vi "Test Decimator with State.vi"() -> ()   [LabVIEW 2019, in "DSP.lvclass"]
uses:
  DSP.lvclass
  Decimate DFD (Array).vi/949379ad-8373-41eb-be01-93a6c1c1afb3.vi
  Decimate DFD (Array).vi/efb08f77-0c38-4651-8a9c-351b9595fc15.vi
  <vilib>/addons/_JKI Toolkits/Caraya/classes/Assert/Assert Equal Value_Variant.vi
  <vilib>/addons/_JKI Toolkits/Caraya/classes/Assert/Assert.lvclass
  <vilib>/addons/_JKI Toolkits/Caraya/classes/Test/Test.lvclass
panel:
  out "Y":dbl[](array[numeric])
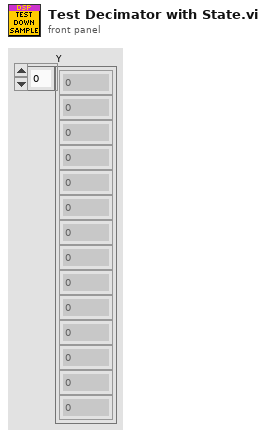
[diagram p1: front panel]
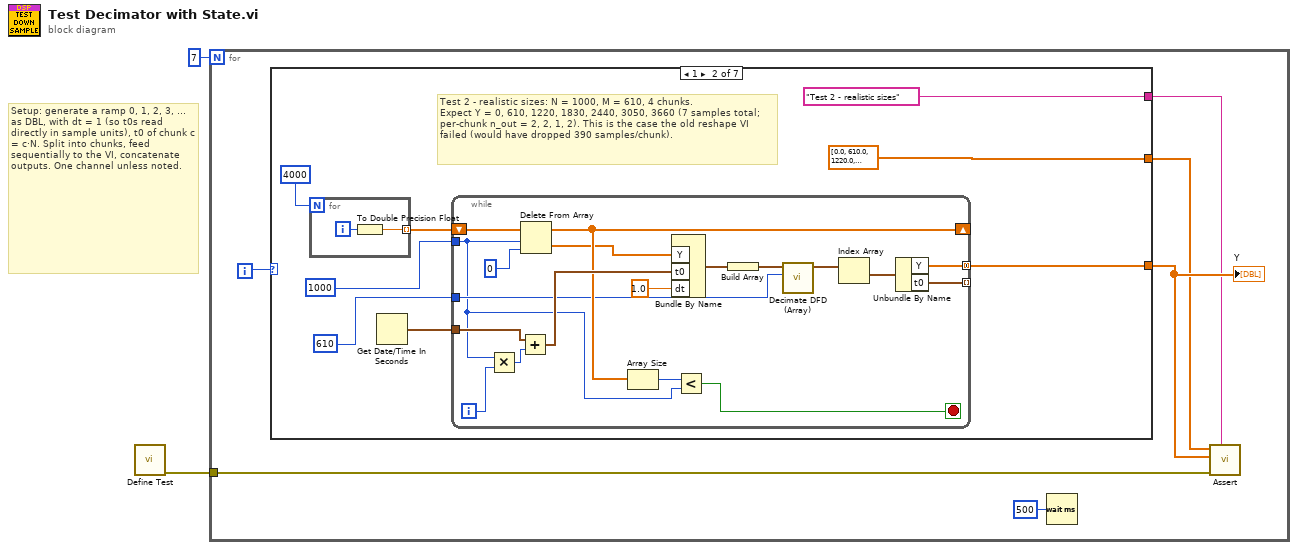
[diagram p0: block diagram]
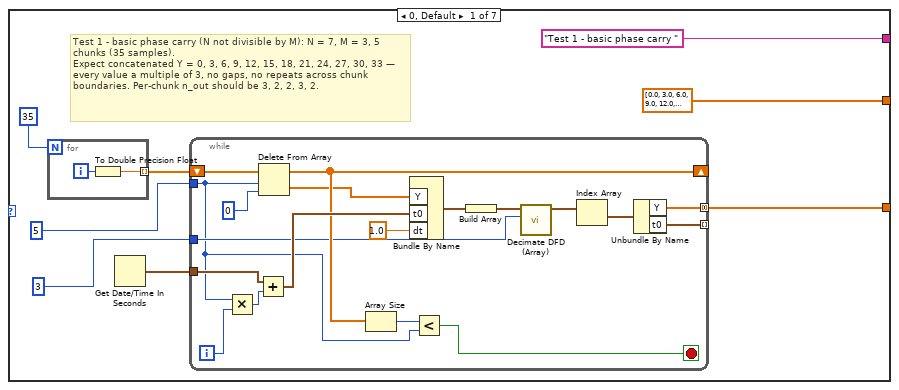
[diagram p2: hidden frame]
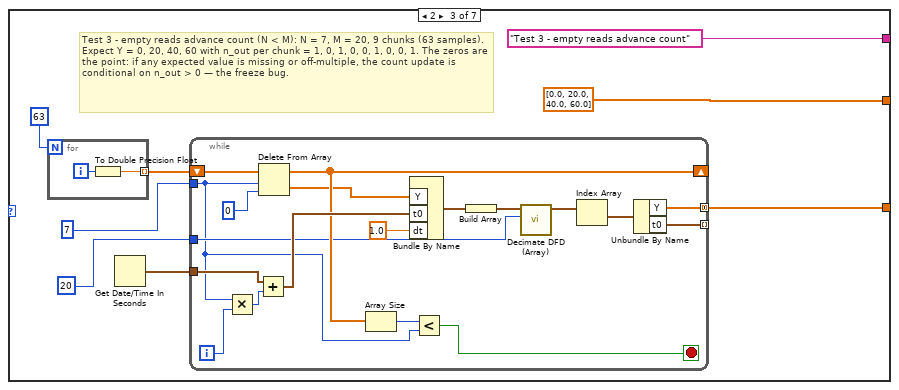
[diagram p3: hidden frame]
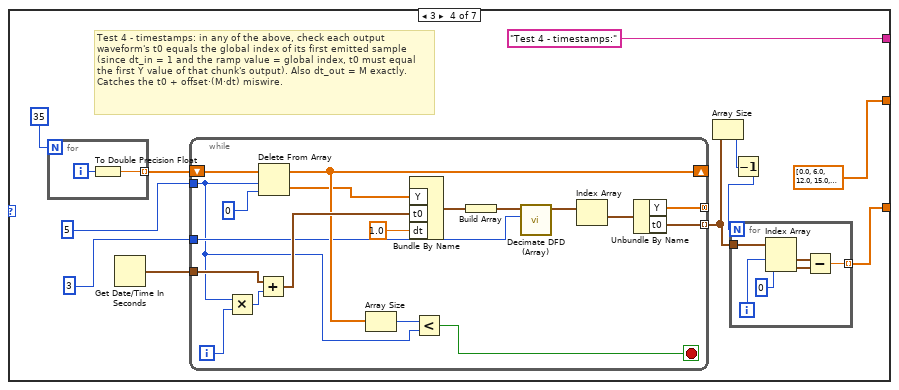
[diagram p4: hidden frame]
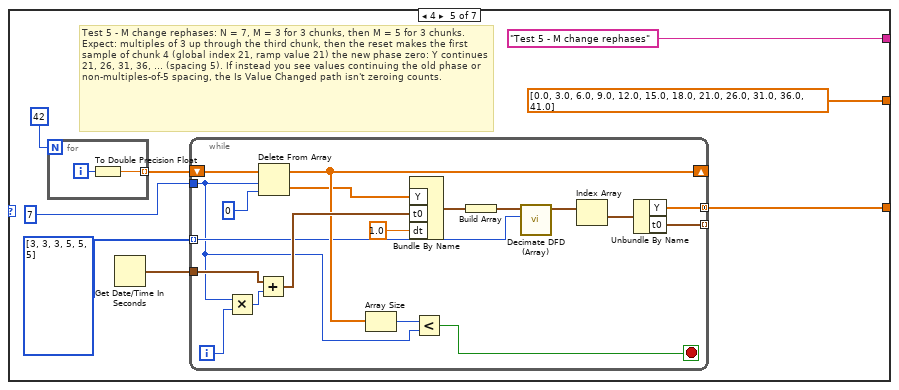
[diagram p5: hidden frame]
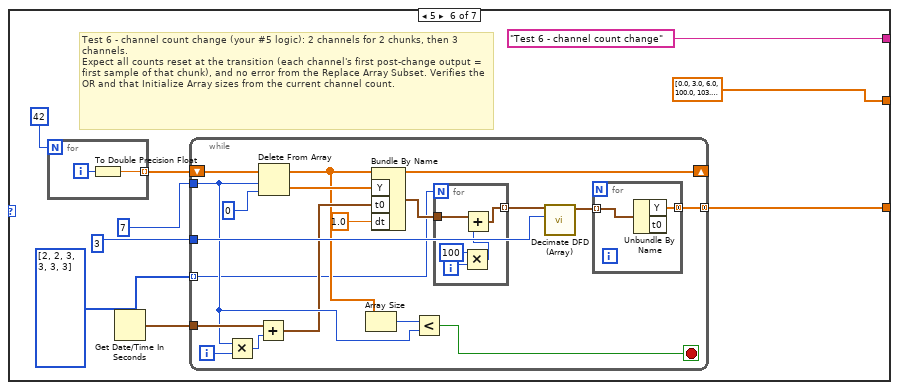
[diagram p6: hidden frame]
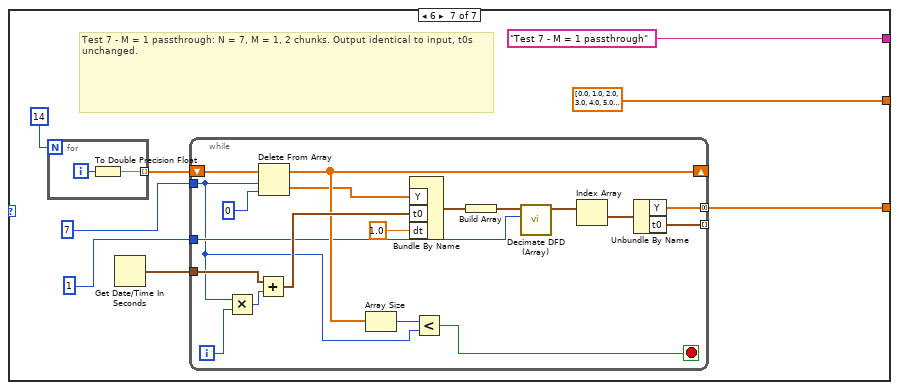
[diagram p7: hidden frame]
diagram:
  # "Setup: generate a ramp 0, 1, 2, 3, … as DBL, with dt = 1 (so t0s read directly in sample units), t0 of chunk c = c·N. Split into chunks, feed sequentially to the VI, concatenate outputs. One channel unless noted."
  n1 = call <vilib>:"Define Test.vi"() -> ("error out"=w1:errorcluster)  [unwired: 10 in, 1 out]
  n2 = for {
    N: 7 -> [_]
    tunnel: w1 -> [w4]
    i -> [w8]
    n3 = case shown="1" w8 {
      tunnel: [w16 w45 w74 w96 w141 w163 w206] -> w7
      tunnel: [dbl[] [0.0, 3.0, 6.0, 9.0, 12.0, 15.0, 18.0, 21.0, 24.0, 27.0, 30.0, 33.0] ("Y 2") dbl[] [0.0, 610.0, 1220.0, 1830.0, 2440.0, 3050.0, 3660.0] ("Y 2") dbl[] [0.0, 20.0, 40.0, 60.0] ("Y 2") dbl[] [0.0, 6.0, 12.0, 15.0, 21.0, 27.0] ("Array 2") dbl[] [0.0, 3.0, 6.0, 9.0, 12.0, 15.0, 18.0, 21.0, 26.0, 31.0, 36.0, 41.0] ("Y 2") dbl[] [0.0, 3.0, 6.0, 100.0, 103.0, 106.0, 9.0, 12.0, 109.0, 112.0, 14.0, 17.0, 20.0, 114.0, 117.0, 120.0, 214.0, 217.0, 220.0, 23.0, 26.0, 123.0, 126.0, 223.0, 226.0, 29.0, 32.0, 129.0, 132.0, 229.0, 232.0, 35.0, 38.0, 41.0, 135.0, 138.0, 141.0, 235.0, 238.0, 241.0] ("Y 3") dbl[] [0.0, 1.0, 2.0, 3.0, 4.0, 5.0, 6.0, 7.0, 8.0, 9.0, 10.0, 11.0, 12.0, 13.0] ("Y 2")] -> w6
      tunnel: ["Test 1 - basic phase carry " "Test 2 - realistic sizes" "Test 3 - empty reads advance count" "Test 4 - timestamps:" "Test 5 - M change rephases" "Test 6 - channel count change" "Test 7 - M = 1 passthrough"] -> w5
      frame 0, Default {
        # "Test 1 - basic phase carry (N not divisible by M): N = 7, M = 3, 5 chunks (35 samples).\nExpect concatenated Y = 0, 3, 6, 9, 12, 15, 18, 21, 24, 27, 30, 33 — every value a multiple of 3, no gaps, no repeats across chunk boundaries. Per-chunk n_out should be 3, 2, 2, 3, 2."
        n4 = for {
          N: 35 ("samples") -> [_]
          tunnel: [w36] -> w15 mode=indexing
          i -> [w37]
          n5 = To Double Precision Float(number=w37) -> (double precision float=w36:dbl)
        }
        n6 = Get Date/Time In Seconds() -> (seconds since 1Jan1904=w14:timestamp)
        n7 = while {
          tunnel: [w32] -> w16 mode=concatenating
          shift-right: [w21] -> _
          shift-left: w15 -> [w30]
          tunnel: 5 ("N") -> [w17]
          tunnel: w14 -> [w23]
          tunnel: 3 ("M") -> [w19]
          tunnel: [w18] -> _ mode=indexing
          i -> [w25]
          stop <- w27 stop-if-true
          n8 = Multiply(x=w17, y=w25) -> (x*y=w24:i32)
          n9 = Add(x=w23, y=w24) -> (x+y=w22:timestamp)
          n10 = Delete From Array(array=w30, length=w17, index=0) -> (deleted portion=w20:dbl[], array with subset deleted=w21:dbl[])
          n11 = Array Size(array=w21) -> (size(s)=w28:i32)
          n12 = Bundle By Name("Y"=w20, "t0"=w22, "dt"=1.0) -> (w26:waveform(dbl))  [unwired: 1 in]
          n13 = Less?(x=w28, y=w17) -> (x < y?=w27:bool)
          n14 = Build Array(w26) -> (w35:waveform(dbl)[])
          n15 = call "Decimate DFD (Array).vi"("Decimation Factor"=w19, "Waveforms in"=w35) -> ("waveforms out"=w34:waveform(dbl)[])  [unwired: 8 in, 1 out]
          n16 = Index Array(array=w34) -> (element=w33:waveform(dbl))  [unwired: 1 in]
          n17 = Unbundle By Name(w33) -> ("Y"=w32:dbl[], "t0"=w18:timestamp)
        }
      }
      frame 1 {
        # "Test 2 - realistic sizes: N = 1000, M = 610, 4 chunks.\nExpect Y = 0, 610, 1220, 1830, 2440, 3050, 3660 (7 samples total; per-chunk n_out = 2, 2, 1, 2). This is the case the old reshape VI failed (would have dropped 390 samples/chunk)."
        n18 = for {
          N: 4000 ("samples") -> [_]
          tunnel: [w65] -> w44 mode=indexing
          i -> [w66]
          n19 = To Double Precision Float(number=w66) -> (double precision float=w65:dbl)
        }
        n20 = Get Date/Time In Seconds() -> (seconds since 1Jan1904=w43:timestamp)
        n21 = while {
          tunnel: [w61] -> w45 mode=concatenating
          shift-right: [w50] -> _
          shift-left: w44 -> [w59]
          tunnel: 1000 ("N") -> [w46]
          tunnel: w43 -> [w52]
          tunnel: 610 ("M") -> [w48]
          tunnel: [w47] -> _ mode=indexing
          i -> [w54]
          stop <- w56 stop-if-true
          n22 = Multiply(x=w46, y=w54) -> (x*y=w53:i32)
          n23 = Add(x=w52, y=w53) -> (x+y=w51:timestamp)
          n24 = Delete From Array(array=w59, length=w46, index=0) -> (deleted portion=w49:dbl[], array with subset deleted=w50:dbl[])
          n25 = Array Size(array=w50) -> (size(s)=w57:i32)
          n26 = Bundle By Name("Y"=w49, "t0"=w51, "dt"=1.0) -> (w55:waveform(dbl))  [unwired: 1 in]
          n27 = Less?(x=w57, y=w46) -> (x < y?=w56:bool)
          n28 = Build Array(w55) -> (w64:waveform(dbl)[])
          n29 = call "Decimate DFD (Array).vi"("Decimation Factor"=w48, "Waveforms in"=w64) -> ("waveforms out"=w63:waveform(dbl)[])  [unwired: 8 in, 1 out]
          n30 = Index Array(array=w63) -> (element=w62:waveform(dbl))  [unwired: 1 in]
          n31 = Unbundle By Name(w62) -> ("Y"=w61:dbl[], "t0"=w47:timestamp)
        }
      }
      frame 2 {
        # "Test 3 - empty reads advance count (N < M): N = 7, M = 20, 9 chunks (63 samples).\nExpect Y = 0, 20, 40, 60 with n_out per chunk = 1, 0, 1, 0, 0, 1, 0, 0, 1. The zeros are the point: if any expected value is missing or off-multiple, the count update is conditional on n_out > 0 — the freeze bug."
        n32 = for {
          N: 63 ("samples") -> [_]
          tunnel: [w94] -> w73 mode=indexing
          i -> [w95]
          n33 = To Double Precision Float(number=w95) -> (double precision float=w94:dbl)
        }
        n34 = Get Date/Time In Seconds() -> (seconds since 1Jan1904=w72:timestamp)
        n35 = while {
          tunnel: [w90] -> w74 mode=concatenating
          shift-right: [w79] -> _
          shift-left: w73 -> [w88]
          tunnel: 7 ("N") -> [w75]
          tunnel: w72 -> [w81]
          tunnel: 20 ("M") -> [w77]
          tunnel: [w76] -> _ mode=indexing
          i -> [w83]
          stop <- w85 stop-if-true
          n36 = Multiply(x=w75, y=w83) -> (x*y=w82:i32)
          n37 = Add(x=w81, y=w82) -> (x+y=w80:timestamp)
          n38 = Delete From Array(array=w88, length=w75, index=0) -> (deleted portion=w78:dbl[], array with subset deleted=w79:dbl[])
          n39 = Array Size(array=w79) -> (size(s)=w86:i32)
          n40 = Bundle By Name("Y"=w78, "t0"=w80, "dt"=1.0) -> (w84:waveform(dbl))  [unwired: 1 in]
          n41 = Less?(x=w86, y=w75) -> (x < y?=w85:bool)
          n42 = Build Array(w84) -> (w93:waveform(dbl)[])
          n43 = call "Decimate DFD (Array).vi"("Decimation Factor"=w77, "Waveforms in"=w93) -> ("waveforms out"=w92:waveform(dbl)[])  [unwired: 8 in, 1 out]
          n44 = Index Array(array=w92) -> (element=w91:waveform(dbl))  [unwired: 1 in]
          n45 = Unbundle By Name(w91) -> ("Y"=w90:dbl[], "t0"=w76:timestamp)
        }
      }
      frame 3 {
        # "Test 4 - timestamps: in any of the above, check each output waveform's t0 equals the global index of its first emitted sample (since dt_in = 1 and the ramp value = global index, t0 must equal the first Y value of that chunk's output). Also dt_out = M exactly. Catches the t0 + offset·(M·dt) miswire."
        n46 = for {
          N: 35 ("samples") -> [_]
          tunnel: [w132] -> w106 mode=indexing
          i -> [w133]
          n47 = To Double Precision Float(number=w133) -> (double precision float=w132:dbl)
        }
        n48 = Get Date/Time In Seconds() -> (seconds since 1Jan1904=w105:timestamp)
        n49 = while {
          tunnel: [w128] -> _ mode=concatenating
          shift-right: [w117] -> _
          shift-left: w106 -> [w126]
          tunnel: 5 ("N") -> [w113]
          tunnel: w105 -> [w119]
          tunnel: 3 ("M") -> [w115]
          tunnel: [w114] -> w100 mode=indexing
          i -> [w121]
          stop <- w123 stop-if-true
          n50 = Multiply(x=w113, y=w121) -> (x*y=w120:i32)
          n51 = Add(x=w119, y=w120) -> (x+y=w118:timestamp)
          n52 = Delete From Array(array=w126, length=w113, index=0) -> (deleted portion=w116:dbl[], array with subset deleted=w117:dbl[])
          n53 = Array Size(array=w117) -> (size(s)=w124:i32)
          n54 = Bundle By Name("Y"=w116, "t0"=w118, "dt"=1.0) -> (w122:waveform(dbl))  [unwired: 1 in]
          n55 = Less?(x=w124, y=w113) -> (x < y?=w123:bool)
          n56 = Build Array(w122) -> (w131:waveform(dbl)[])
          n57 = call "Decimate DFD (Array).vi"("Decimation Factor"=w115, "Waveforms in"=w131) -> ("waveforms out"=w130:waveform(dbl)[])  [unwired: 8 in, 1 out]
          n58 = Index Array(array=w130) -> (element=w129:waveform(dbl))  [unwired: 1 in]
          n59 = Unbundle By Name(w129) -> ("Y"=w128:dbl[], "t0"=w114:timestamp)
        }
        n60 = Array Size(array=w100) -> (size(s)=w99:i32)
        n61 = Decrement(x=w99) -> (x-1=w98:i32)
        n62 = for {
          N: w98 -> [_]
          tunnel: w100 -> [w112]
          tunnel: [w109] -> w96 mode=indexing
          i -> [w108]
          n63 = Index Array(array=w112, index #1=w108, index #2=0 ("index")) -> (element #1=w111:timestamp, element #2=w110:timestamp)
          n64 = Subtract(x=w111, y=w110) -> (x-y=w109:dbl)
        }
      }
      frame 4 {
        # "Test 5 - M change rephases: N = 7, M = 3 for 3 chunks, then M = 5 for 3 chunks.\nExpect: multiples of 3 up through the third chunk, then the reset makes the first sample of chunk 4 (global index 21, ramp value 21) the new phase zero: Y continues 21, 26, 31, 36, … (spacing 5). If instead you see values continuing the old phase or non-multiples-of-5 spacing, the Is Value Changed path isn't zeroing counts."
        n65 = for {
          N: 42 ("samples") -> [_]
          tunnel: [w161] -> w140 mode=indexing
          i -> [w162]
          n66 = To Double Precision Float(number=w162) -> (double precision float=w161:dbl)
        }
        n67 = Get Date/Time In Seconds() -> (seconds since 1Jan1904=w139:timestamp)
        n68 = while {
          tunnel: [w157] -> w141 mode=concatenating
          shift-right: [w146] -> _
          shift-left: w140 -> [w155]
          tunnel: 7 ("N") -> [w142]
          tunnel: w139 -> [w148]
          tunnel: i32[] [3, 3, 3, 5, 5, 5] ("M") -> [w144] mode=indexing
          tunnel: [w143] -> _ mode=indexing
          i -> [w150]
          stop <- w152 stop-if-true
          n69 = Multiply(x=w142, y=w150) -> (x*y=w149:i32)
          n70 = Add(x=w148, y=w149) -> (x+y=w147:timestamp)
          n71 = Delete From Array(array=w155, length=w142, index=0) -> (deleted portion=w145:dbl[], array with subset deleted=w146:dbl[])
          n72 = Array Size(array=w146) -> (size(s)=w153:i32)
          n73 = Bundle By Name("Y"=w145, "t0"=w147, "dt"=1.0) -> (w151:waveform(dbl))  [unwired: 1 in]
          n74 = Less?(x=w153, y=w142) -> (x < y?=w152:bool)
          n75 = Build Array(w151) -> (w160:waveform(dbl)[])
          n76 = call "Decimate DFD (Array).vi"("Decimation Factor"=w144, "Waveforms in"=w160) -> ("waveforms out"=w159:waveform(dbl)[])  [unwired: 8 in, 1 out]
          n77 = Index Array(array=w159) -> (element=w158:waveform(dbl))  [unwired: 1 in]
          n78 = Unbundle By Name(w158) -> ("Y"=w157:dbl[], "t0"=w143:timestamp)
        }
      }
      frame 5 {
        # "Test 6 - channel count change (your #5 logic): 2 channels for 2 chunks, then 3 channels.\nExpect all counts reset at the transition (each channel's first post-change output = first sample of that chunk), and no error from the Replace Array Subset. Verifies the OR and that Initialize Array sizes from the current channel count."
        n79 = for {
          N: 42 ("samples") -> [_]
          tunnel: [w197] -> w171 mode=indexing
          i -> [w198]
          n80 = To Double Precision Float(number=w198) -> (double precision float=w197:dbl)
        }
        n81 = Get Date/Time In Seconds() -> (seconds since 1Jan1904=w170:timestamp)
        n82 = while {
          tunnel: [w189] -> w163 mode=concatenating
          shift-right: [w176] -> _
          shift-left: w171 -> [w187]
          tunnel: 7 ("N") -> [w178]
          tunnel: w170 -> [w181]
          tunnel: 3 ("M") -> [w179]
          tunnel: i32[] [2, 2, 3, 3, 3, 3] ("dimension size") -> [w174] mode=indexing
          i -> [w183]
          stop <- w184 stop-if-true
          n83 = Multiply(x=w178, y=w183) -> (x*y=w182:i32)
          n84 = Add(x=w181, y=w182) -> (x+y=w177:timestamp)
          n85 = Delete From Array(array=w187, length=w178, index=0) -> (deleted portion=w180:dbl[], array with subset deleted=w176:dbl[])
          n86 = Array Size(array=w176) -> (size(s)=w185:i32)
          n87 = Bundle By Name("Y"=w180, "t0"=w177, "dt"=1.0) -> (w175:waveform(dbl))  [unwired: 1 in]
          n88 = Less?(x=w185, y=w178) -> (x < y?=w184:bool)
          n89 = for {
            N: w174 -> [_]
            tunnel: w175 -> [w196]
            tunnel: [w192] -> w173 mode=indexing
            i -> [w195]
            n90 = Multiply(x=100, y=w195) -> (x*y=w193:i32)
            n91 = Add(x=w196, y=w193) -> (x+y=w192:waveform(dbl))
          }
          n92 = call "Decimate DFD (Array).vi"("Decimation Factor"=w179, "Waveforms in"=w173) -> ("waveforms out"=w172:waveform(dbl)[])  [unwired: 8 in, 1 out]
          n93 = for {
            tunnel: [w191] -> w189 mode=concatenating
            tunnel: w172 -> [w190] mode=indexing
            n94 = Unbundle By Name(w190) -> ("Y"=w191:dbl[])  [unwired: 1 out]
          }
        }
      }
      frame 6 {
        # "Test 7 - M = 1 passthrough: N = 7, M = 1, 2 chunks. Output identical to input, t0s unchanged."
        n95 = for {
          N: 14 ("samples") -> [_]
          tunnel: [w226] -> w205 mode=indexing
          i -> [w227]
          n96 = To Double Precision Float(number=w227) -> (double precision float=w226:dbl)
        }
        n97 = Get Date/Time In Seconds() -> (seconds since 1Jan1904=w204:timestamp)
        n98 = while {
          tunnel: [w222] -> w206 mode=concatenating
          shift-right: [w211] -> _
          shift-left: w205 -> [w220]
          tunnel: 7 ("N") -> [w207]
          tunnel: w204 -> [w213]
          tunnel: 1 ("M") -> [w209]
          tunnel: [w208] -> _ mode=indexing
          i -> [w215]
          stop <- w217 stop-if-true
          n99 = Multiply(x=w207, y=w215) -> (x*y=w214:i32)
          n100 = Add(x=w213, y=w214) -> (x+y=w212:timestamp)
          n101 = Delete From Array(array=w220, length=w207, index=0) -> (deleted portion=w210:dbl[], array with subset deleted=w211:dbl[])
          n102 = Array Size(array=w211) -> (size(s)=w218:i32)
          n103 = Bundle By Name("Y"=w210, "t0"=w212, "dt"=1.0) -> (w216:waveform(dbl))  [unwired: 1 in]
          n104 = Less?(x=w218, y=w207) -> (x < y?=w217:bool)
          n105 = Build Array(w216) -> (w225:waveform(dbl)[])
          n106 = call "Decimate DFD (Array).vi"("Decimation Factor"=w209, "Waveforms in"=w225) -> ("waveforms out"=w224:waveform(dbl)[])  [unwired: 8 in, 1 out]
          n107 = Index Array(array=w224) -> (element=w223:waveform(dbl))  [unwired: 1 in]
          n108 = Unbundle By Name(w223) -> ("Y"=w222:dbl[], "t0"=w208:timestamp)
        }
      }
    }
    "Y" <- w7
    n109 = Wait (ms)(milliseconds to wait=u32 500) -> ()  [unwired: 1 out]
    n110 = call-poly <vilib>:"Assert.vi"("Label"=w5, "error in (no error)"=w4, "Actual"=w7, "Expected"=w6) -> ()  [unwired: 6 in, 2 out]
  }
